vi "CALIBRATION_SUMMARY.vi"(0 "flow_slope_IN":dbl=50.0 format="%.2f", 1 "flow_slope_OUT":dbl=56.0 format="%.2f", 2 "Path":path=path "C:/KPRO_2010/Output_files/slopes-cal-record.txt", 3 "pressure_slope_OUT":dbl=23.33 format="%.2f", 5 "pressure_slope_IN":dbl=23.33 format="%.2f", 9 "string_pot_slope_IN":dbl=1.5 format="%.2f", 11 "error in (no error)":errorcluster, 12 "string_pot_slope_OUT":dbl=1.5 format="%.2f") -> (15 "error out":errorcluster)   [LabVIEW 2016]
uses:
  <vilib>/Utility/file.llb/Write Delimited Spreadsheet (string).vi
  C/Program Files (x86)/National Instruments/LabVIEW 2016/user.lib/_OpenG.lib/file/file.llb/Strip Path - Traditional__ogtk.vi
  Kpro Globals.vi
  C/Program Files (x86)/National Instruments/LabVIEW 2016/user.lib/_OpenG.lib/file/file.llb/Build Path - Traditional__ogtk.vi
  <vilib>/Utility/file.llb/Write Delimited Spreadsheet (DBL).vi
panel:
  out "KPRO Box Number":dbl=800.0
  out "Date_and_time":string
  out "pressure_slope_OUT 2":dbl=23.33 format="%.2f"
  out "flow_slope_OUT 2":dbl=51.35 format="%.2f"
  out "string_pot_slope_OUT 2":dbl=1.5 format="%.2f"
  out "pressure_slope_IN 2":dbl=23.33 format="%.2f"
  out "flow_slope_IN 2":dbl=51.35 format="%.2f"
  out "string_pot_slope_IN 2":dbl=1.5 format="%.2f"
  in  "ok":bool
  # "CALIBRATION SUMMARY"
  # "Record these values in Kpro Box Calibration Log"
  # "DATE"
  # "TIME"
  # "Initial Slope              New Slope"
  # "Flow Sensor"
  # "Pressure Transducer"
  # "String Potentiometer"
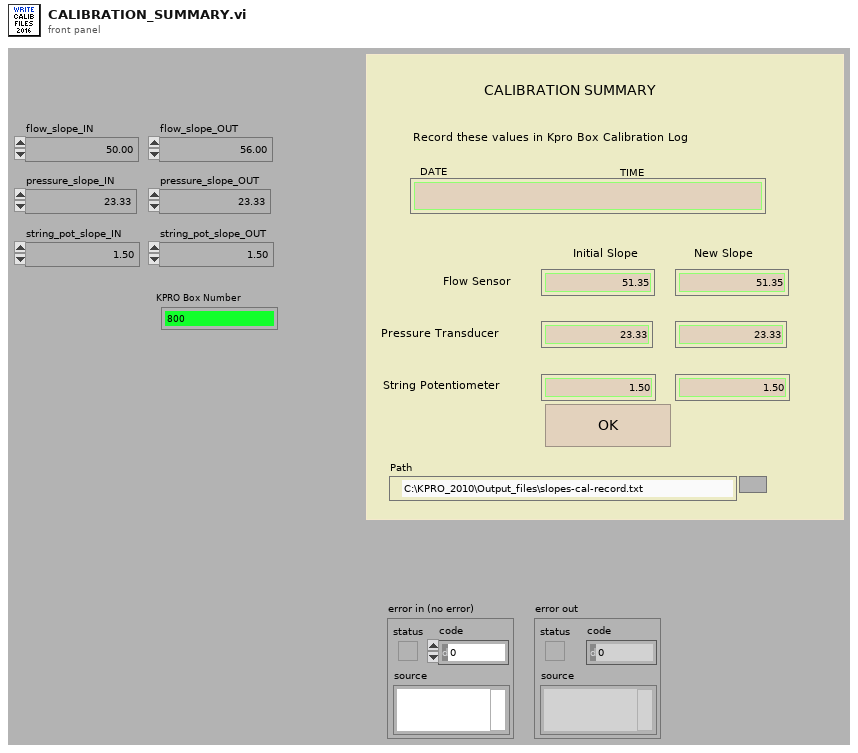
[diagram p1: front panel]
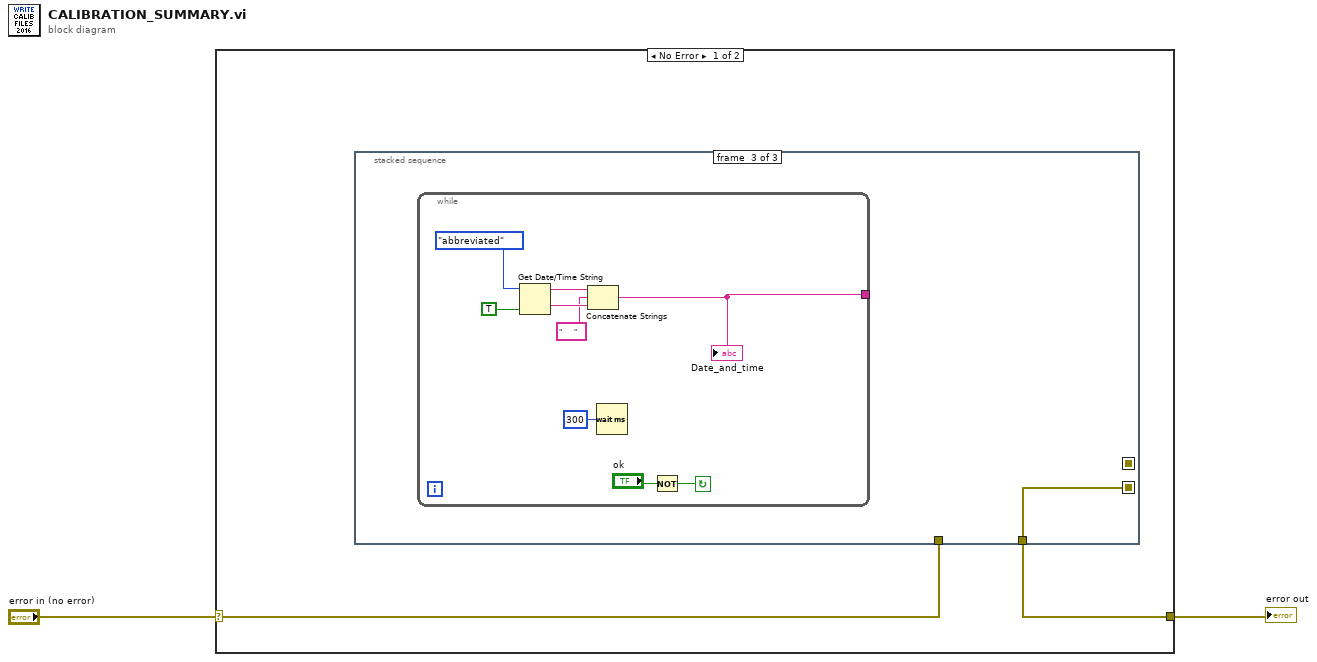
[diagram p0: block diagram]
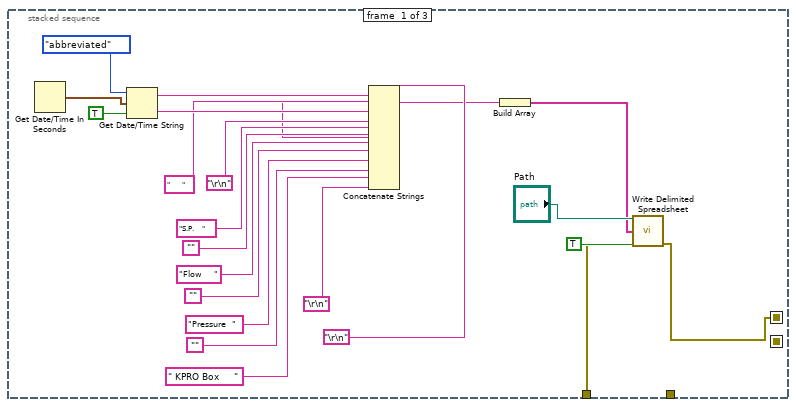
[diagram p2: hidden frame]
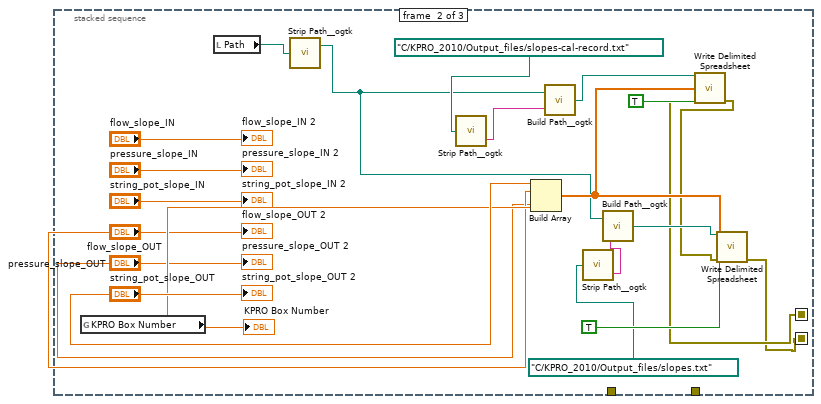
[diagram p3: hidden frame]
diagram:
  n1 = case shown="No Error" "error in (no error)" {
    selector: "error in (no error)" -> [w4 w58]
    tunnel: [w3 w58] -> w2
    frame No Error {
      n2 = stacked-sequence {
        seq-local: [w5 _ _] -> [_ w28 _]
        seq-local: [_ w27 _] -> [_ _ w48]
        tunnel: w4 -> [w9 _ _]
        tunnel: [_ _ w48] -> w3
        frame #0 {
          n3 = Get Date/Time In Seconds() -> (seconds since 1Jan1904=w6:timestamp)
          n4 = Get Date/Time String(date format (0)=enum16{"short", "long", "abbreviated"}."abbreviated", seconds (now)=w6, want seconds? (F)=TRUE) -> (date string=w22:string, time string=w21:string)
          n5 = Concatenate Strings("\r\n", w22, "      " ("string"), w21, "\r\n", "S.P.    " ("string"), "" ("string"), "Flow    " ("string"), "" ("string"), "Pressure  " ("string"), "" ("string"), " KPRO Box     " ("string"), "\r\n") -> (w8:string)
          n6 = Build Array(w8) -> (w7:string[])
          n7 = call-poly <vilib>:"Write Delimited Spreadsheet.vi"("file path (dialog if empty)"="Path", "1D data"=w7, "append to file? (new file:F)"=TRUE, "error in (no error)"=w9) -> ("error out"=w5:errorcluster)  [unwired: 10 in, 1 out]
        }
        frame #1 {
          n8 = global read "Kpro Globals.vi" "KPRO Box Number"() -> (w40:dbl)
          "KPRO Box Number" <- w40
          n9 = local read "Path"() -> (w37:path)
          n10 = call-poly "Strip Path__ogtk.vi"("path"=w37) -> ("stripped path"=w32:path)  [unwired: 1 out]
          n11 = call-poly "Strip Path__ogtk.vi"("path"=path "C:/KPRO_2010/Output_files/slopes-cal-record.txt") -> ("name"=w35:string)  [unwired: 1 out]
          n12 = Build Array("string_pot_slope_OUT", "flow_slope_OUT", "pressure_slope_OUT", w40) -> (w41:dbl[])
          n13 = call-poly "Build Path__ogtk.vi"("name or relative path"=w35, "base path"=w32) -> ("appended path"=w34:path)
          n14 = call-poly "Strip Path__ogtk.vi"("path"=path "C:/KPRO_2010/Output_files/slopes.txt") -> ("name"=w31:string)  [unwired: 1 out]
          n15 = call-poly "Build Path__ogtk.vi"("name or relative path"=w31, "base path"=w32) -> ("appended path"=w30:path)
          n16 = call-poly <vilib>:"Write Delimited Spreadsheet.vi"("file path (dialog if empty)"=w34, "1D data"=w41, "append to file? (new file:F)"=TRUE, "error in (no error)"=w28) -> ("error out"=w29:errorcluster)  [unwired: 10 in, 1 out]
          n17 = call-poly <vilib>:"Write Delimited Spreadsheet.vi"("file path (dialog if empty)"=w30, "1D data"=w41, "append to file? (new file:F)"=TRUE, "error in (no error)"=w29) -> ("error out"=w27:errorcluster)  [unwired: 10 in, 1 out]
          "pressure_slope_IN 2" <- "pressure_slope_IN"
          "flow_slope_IN 2" <- "flow_slope_IN"
          "string_pot_slope_IN 2" <- "string_pot_slope_IN"
          "pressure_slope_OUT 2" <- "pressure_slope_OUT"
          "flow_slope_OUT 2" <- "flow_slope_OUT"
          "string_pot_slope_OUT 2" <- "string_pot_slope_OUT"
        }
        frame #2 {
          n18 = while {
            tunnel: [w49] -> _
            stop <- w57 continue-if-true
            n19 = Get Date/Time String(date format (0)=enum16{"short", "long", "abbreviated"}."abbreviated", want seconds? (F)=TRUE) -> (date string=w54:string, time string=w51:string)  [unwired: 1 in]
            n20 = Concatenate Strings(w54, "      " ("string"), w51) -> (w49:string)
            "Date_and_time" <- w49
            n21 = Wait (ms)(milliseconds to wait=u32 300) -> ()  [unwired: 1 out]
            n22 = Not(x="ok") -> (.not. x?=w57:bool)
          }
        }
      }
    }
    frame Error {
    }
  }
  "error out" <- w2
